vi "Temperature Warnings.vi"(8 "Error In":errorcluster, 11 "Weather Data In":T1={"Current Temperature"=0.0, "Max Temperature"=0.0, "Min Temperature"=0.0, "Temperature Warning Text"="No Warning", "Temperature Warning?"=FALSE, "Current Windspeed"=0.0, "Max Windspeed"=0.0, "Windspeed Warning?"=FALSE, "Windspeed Warning Text"=""}) -> (0 "Error Out":errorcluster, 3 "Weather Data Out":T1)   [LabVIEW 2017]
doc: "This VI is used to determine the string to output to the weather station based on the current temperature and limit settings.\n\nInputs: Current Temperature (DBL), Minimum Temperature (DBL), and Maximum Temperature (DBL).\nOutputs: Warning Text (string) and Warning? (Boolean)."
uses:
  Weather Data.ctl
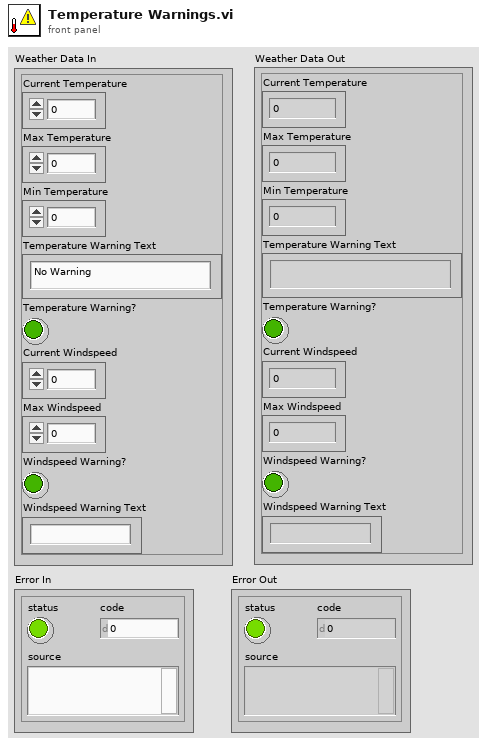
[diagram p1: front panel]
types:
  T1 = typedef "Weather Data.ctl" = cluster{"Current Temperature":dbl, "Max Temperature":dbl, "Min Temperature":dbl, "Temperature Warning Text":string, "Temperature Warning?":bool, "Current Windspeed":dbl, "Max Windspeed":dbl, "Windspeed Warning?":bool, "Windspeed Warning Text":string}
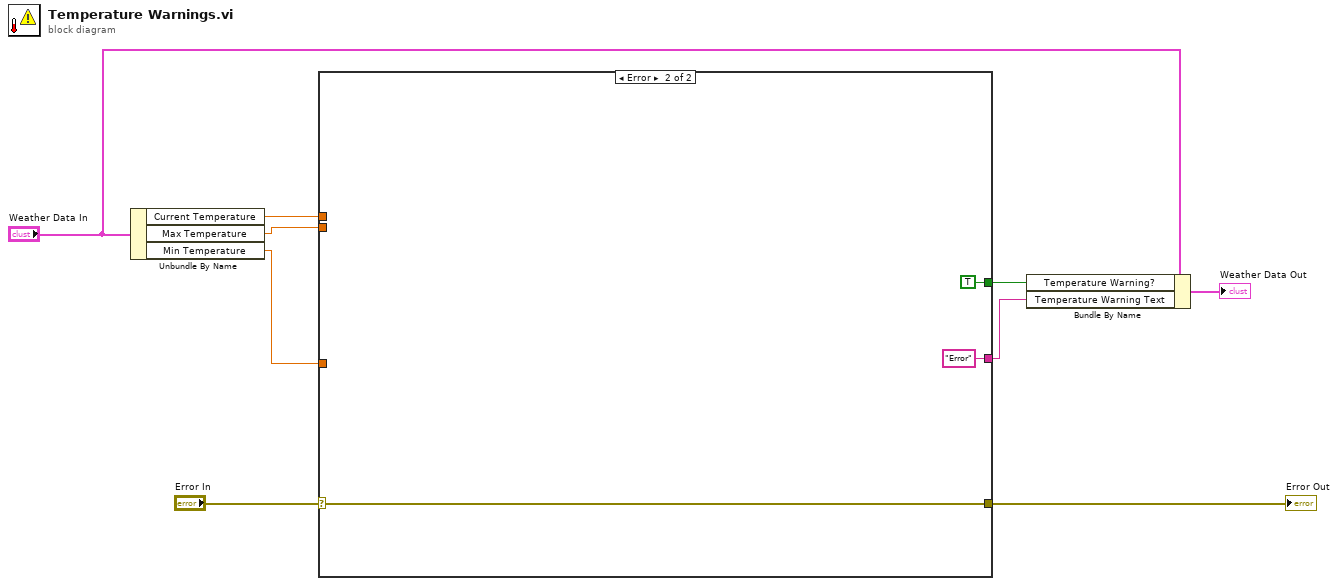
[diagram p0: block diagram]
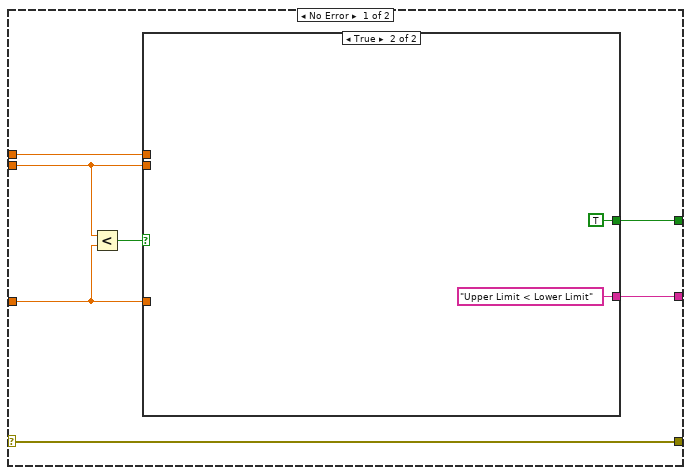
[diagram p2: hidden frame]
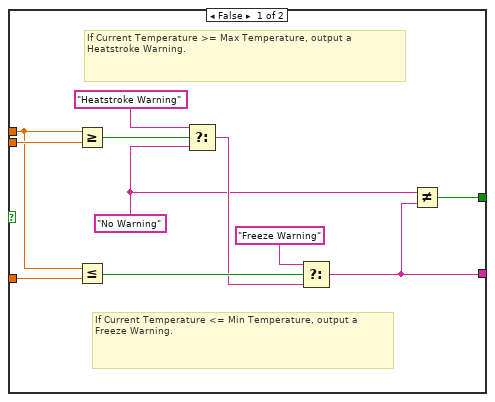
[diagram p3: hidden frame]
diagram:
  n1 = Unbundle By Name("Weather Data In") -> ("Current Temperature"=w8:dbl, "Max Temperature"=w9:dbl, "Min Temperature"=w7:dbl)
  n2 = case shown="Error" "Error In" {
    selector: "Error In" -> [w16 w32]
    tunnel: w9 -> [w11 _]
    tunnel: w8 -> [w13 _]
    tunnel: w7 -> [w10 _]
    tunnel: [w16 w32] -> w5
    tunnel: [w15 TRUE] -> w4
    tunnel: [w14 "Error" ("f")] -> w3
    frame No Error {
      n3 = Less?(x=w11, y=w10) -> (x < y?=w12:bool)
      n4 = case shown="True" w12 {
        tunnel: w11 -> [w21 _]
        tunnel: w10 -> [w20 _]
        tunnel: [w19 TRUE] -> w15
        tunnel: [w18 "Upper Limit < Lower Limit" ("f")] -> w14
        tunnel: w13 -> [w17 _]
        frame False {
          w22 = "No Warning" ("f")
          # "If Current Temperature <= Min Temperature, output a Freeze Warning."
          # "If Current Temperature >= Max Temperature, output a Heatstroke Warning."
          n5 = Greater Or Equal?(x=w17, y=w21) -> (x >= y?=w27:bool)
          n6 = Less Or Equal?(x=w17, y=w20) -> (x <= y?=w24:bool)
          n7 = Select(t="Heatstroke Warning", s=w27, f=w22) -> (s? t:f=w23:string)
          n8 = Select(t="Freeze Warning", s=w24, f=w23) -> (s? t:f=w18:string)
          n9 = Not Equal?(x=w22, y=w18) -> (x != y?=w19:bool)
        }
        frame True {
        }
      }
    }
    frame Error {
    }
  }
  "Error Out" <- w5
  n10 = Bundle By Name(cluster="Weather Data In", "Temperature Warning?"=w4, "Temperature Warning Text"=w3) -> (→"Weather Data Out":T1)
